vi "Enhance Json Config with Channels.vi"(6 "Save PAtools config Json? (Default: True)":bool=TRUE, 8 "error in":errorcluster, 9 "Channels Array":T1[](array[typedef]), 10 "Channels":cluster{"Channels":T1[]}, 11 "Json Config":string="{\"Version\":{\"Major\":2,\"Minor\":0,\"Fix\":0,\"Build\":0},\"Configuration\":{\"Name\":\"Custom Parameters\",\"DataType\":\"Container\",\"ExtraTypeInfo\":\"\",\"DataValue\":\"\",\"SubNodes\":[{\"Name\":\"Common\",\"DataType\":\"Container\",\"ExtraTypeInfo\":\"\",\"DataValue\":\"\",\"SubNodes\":[{\"Name\":\"Iteration Interval (s)\",\"DataType\":\"Double\",\"ExtraTypeInfo\":\"\",\"DataValue\":\"0.001000\",\"SubNodes\":[]},{\"Name\":\"T0 (ns)\",\"DataType\":\"U64\",\"ExtraTypeInfo\":\"\",\"DataValue\":\"0\",\"SubNodes\":[]},{\"Name\":\"Priority\",\"DataType\":\"I32\",\"ExtraTypeInfo\":\"\",\"DataValue\":\"100\",\"SubNodes\":[]},{\"Name\":\"Processor\",\"DataType\":\"I32\",\"ExtraTypeInfo\":\"\",\"DataValue\":\"-2\",\"SubNodes\":[]},{\"Name\":\"Wait in Ready State\",\"DataType\":\"Boolean\",\"ExtraTypeInfo\":\"\",\"DataValue\":\"TRUE\",\"SubNodes\":[]}]},{\"Name\":\"Amount of Channels\",\"DataType\":\"U32\",\"ExtraTypeInfo\":\"\",\"DataValue\":\"0\",\"SubNodes\":[]},{\"Name\":\"Address\",\"DataType\":\"String\",\"ExtraTypeInfo\":\"\",\"DataValue\":\"\",\"SubNodes\":[]}]}}") -> (0 "error out":errorcluster, 3 "PAtools JSON":string)   [LabVIEW 2024, in "Utilities.lvlib"]
uses:
  Utilities.lvlib
  Channel.ctl
  <vilib>/JDP Science/JSONtext/JSONtext.lvlib
panel:
  in  "Name":cluster{"Name":string}
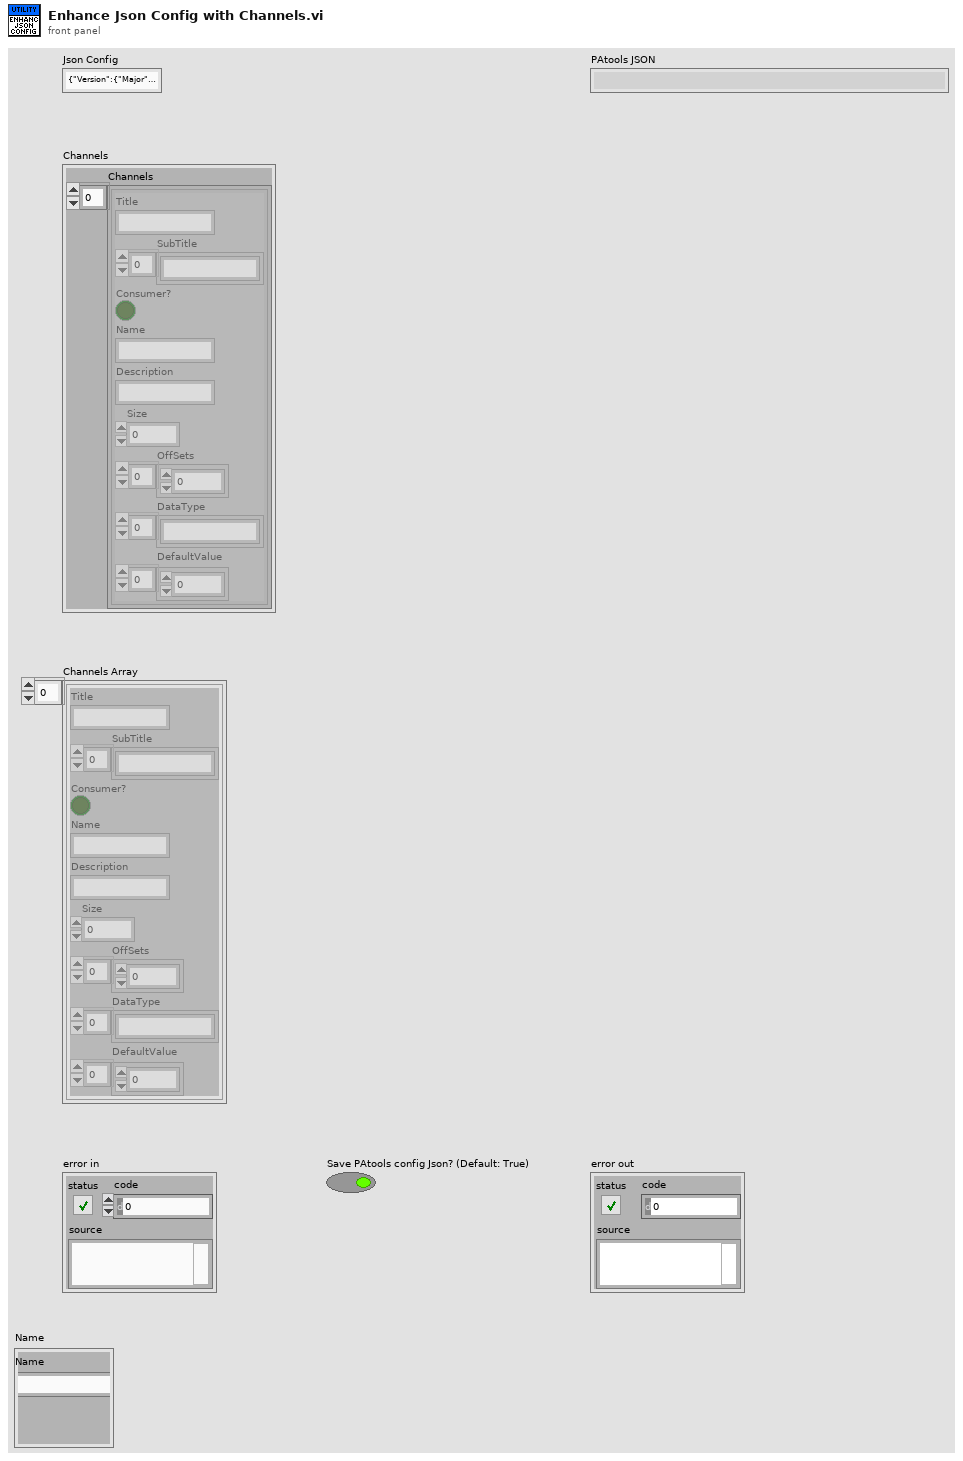
[diagram p1: front panel]
types:
  T1 = typedef "Utilities.lvlib/Channel.ctl" = cluster{"Title":string, "SubTitle":string[], "Consumer?":bool, "Name":string, "Description":string, "Size":i32, "OffSets":i32[], "DataType":string[], "DefaultValue":dbl[]}
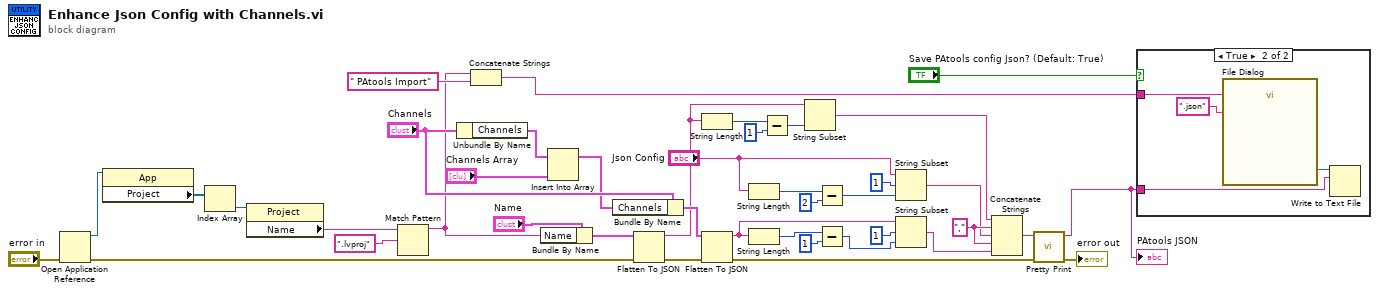
[diagram p0: block diagram]
diagram:
  w40 = "," ("string")
  n1 = Open Application Reference(8:"error in") -> (0:w17:errorcluster, 3:w22:refnum<vi>)  [unwired: 3 in]
  n2 = property class="App"(reference=w22) -> ("Project"=w21:refnum<vi>[])  [unwired: 1 in, 2 out]
  n3 = Index Array(array=w21) -> (element=w20:refnum<vi>)  [unwired: 1 in]
  n4 = property class="Project"(reference=w20) -> ("Name"=w19:string)  [unwired: 1 in, 2 out]
  n5 = Match Pattern(string=w19, regular expression=".lvproj") -> (before substring=w4:string)  [unwired: 1 in, 3 out]
  n6 = Unbundle By Name("Channels") -> ("Channels"=w12:T1[])
  n7 = Concatenate Strings(w4, " PAtools Import" ("string")) -> (w3:string)
  n8 = Bundle By Name(cluster="Name", "Name"=w4) -> (w5:cluster{"Name":string})
  n9 = Insert Into Array(array=w12, new element="Channels Array") -> (w9:T1[])  [unwired: 1 in]
  n10 = Bundle By Name(cluster="Channels", "Channels"=w9) -> (w8:cluster{"Channels":T1[]})
  n11 = Flatten To JSON(anything=w5, error in (no error)=w17) -> (JSON string=w6:string, 11:w16:errorcluster)  [unwired: 1 in]
  n12 = String Length(string=w6) -> (length=w39:i32)
  n13 = Flatten To JSON(anything=w8, error in (no error)=w16) -> (JSON string=w23:string, 11:w15:errorcluster)  [unwired: 1 in]
  n14 = String Length(string="Json Config") -> (length=w35:i32)
  n15 = String Length(string=w23) -> (length=w30:i32)
  n16 = Subtract(x=w39, y=1) -> (x-y=w37:i32)
  n17 = String Subset(string=w6, length (rest)=w37) -> (substring=w36:string)  [unwired: 1 in]
  n18 = Subtract(x=w35, y=2) -> (x-y=w32:i32)
  n19 = Subtract(x=w30, y=1) -> (x-y=w28:i32)
  n20 = String Subset(string="Json Config", offset (0)=1, length (rest)=w32) -> (substring=w31:string)
  n21 = String Subset(string=w23, offset (0)=1, length (rest)=w28) -> (substring=w27:string)
  n22 = Concatenate Strings(w36, w40, w31, w40, w27) -> (w25:string)
  n23 = call <vilib>:"Pretty Print.vi"("error in (no error)"=w15, "JSON"=w25) -> ("error out"=→"error out":errorcluster, "<JSON>"=w2:string)  [unwired: 7 in, 1 out]
  "PAtools JSON" <- w2
  n24 = case shown="True" "Save PAtools config Json? (Default: True)" {
    tunnel: w2 -> [_ w45]
    tunnel: w3 -> [_ w43]
    frame False {
    }
    frame True {
      n25 = call "File Dialog"("default name"=w43, "pattern (all files)"=".json") -> ("selected path"=w44:path)  [unwired: 10 in, 3 out]
      n26 = Write to Text File(file (use dialog)=w44, text=w45) -> ()  [unwired: 2 in, 3 out]
    }
  }
